vi "Read Logging Settings.vi"(8 "error in (no error)":errorcluster, 11 "Logger Configuration in":refnum<class "Logger Configuration.lvclass">) -> (0 "error out":errorcluster, 2 "Logging Settings":T1, 3 "Logger Configuration out":refnum<class "Logger Configuration.lvclass">)   [LabVIEW 2017, in "Logger.lvlib" / "Logger Configuration.lvclass"]
uses:
  Logger Configuration.lvclass
  Logger Configuration.lvclass/Logger Configuration.ctl
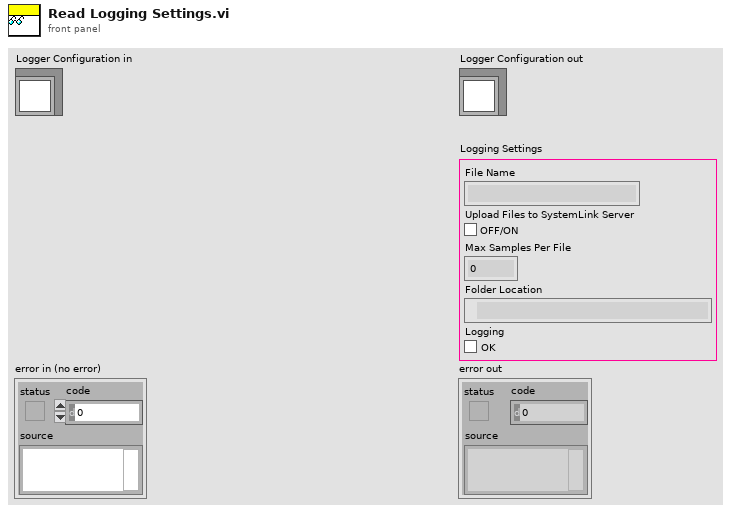
[diagram p1: front panel]
types:
  T1 = cluster{"File Name":string, "Upload Files to SystemLink Server":bool, "Max Samples Per File":i32, "Folder Location":path, "Logging":bool}
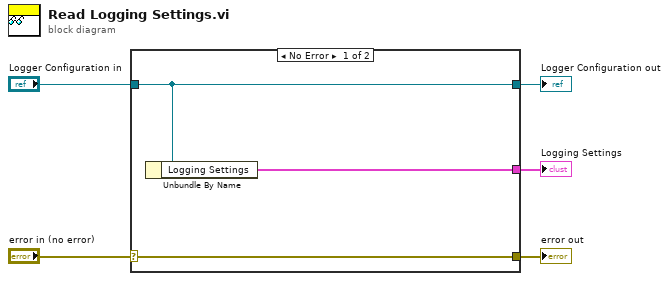
[diagram p0: block diagram]
diagram:
  n1 = case shown="No Error" "error in (no error)" {
    selector: "error in (no error)" -> [w8 w9]
    tunnel: [w8 w9] -> w4
    tunnel: [w7 w10] -> w2
    tunnel: "Logger Configuration in" -> [w7 w10]
    tunnel: [w6 _] -> w1
    frame No Error {
      n2 = Unbundle By Name(w7) -> ("Logging Settings"=w6:T1)
    }
    frame Error {
    }
  }
  "error out" <- w4
  "Logger Configuration out" <- w2
  "Logging Settings" <- w1
